vi "Read channels.vi"(8 "error in (no error)":errorcluster, 11 "String Compare Config in":refnum<class "String Compare Config.lvclass">) -> (0 "error out":errorcluster, 2 "Channels":refnum<class "TBM channel.lvclass">[](array[class]), 3 "String Compare Config out":refnum<class "String Compare Config.lvclass">)   [LabVIEW 2015, in "String Compare Config.lvclass"]
uses:
  String Compare Config.lvclass
  <vilib>/NI/Tag Bus Module Framework/channel/TBM channel.lvclass
  String Compare Config.lvclass/String Compare Config.ctl
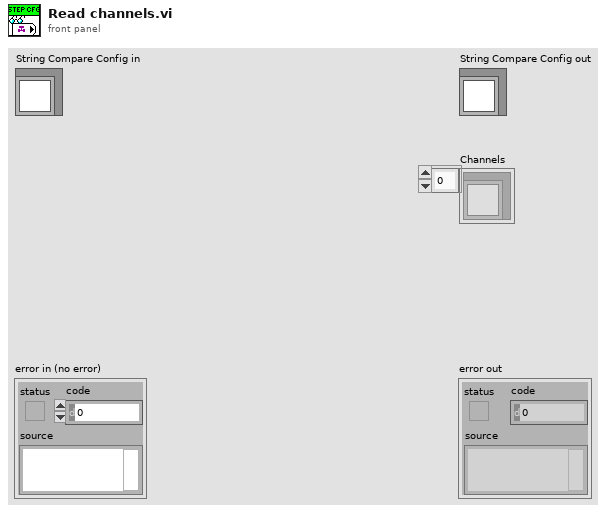
[diagram p1: front panel]
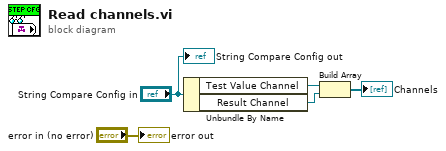
[diagram p0: block diagram]
diagram:
  n1 = Unbundle By Name("String Compare Config in") -> ("Test Value Channel"=w5:refnum<class "TBM channel.lvclass">, "Result Channel"=w4:refnum<class "TBM channel.lvclass">)
  n2 = Build Array(w5, w4) -> (→"Channels":refnum<class "TBM channel.lvclass">[])
  "error out" <- "error in (no error)"
  "String Compare Config out" <- "String Compare Config in"
